vi "fgv_Video Recording Enable.vi"(9 "Function":T1, 11 "Video Recording Enabled":bool) -> (3 "Video Recording Enabled":bool)   [LabVIEW 2013]
uses:
  Typedefs/Read Write Enum.ctl
  Global Variables/General Globals.vi
panel:
  # "SUBROUTINE"
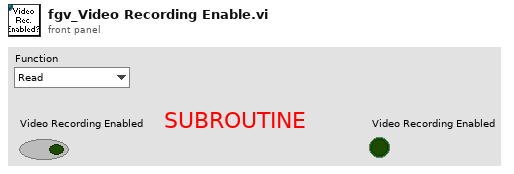
[diagram p1: front panel]
types:
  T1 = typedef "Read Write Enum.ctl" = enum16{"Read", "Write"}
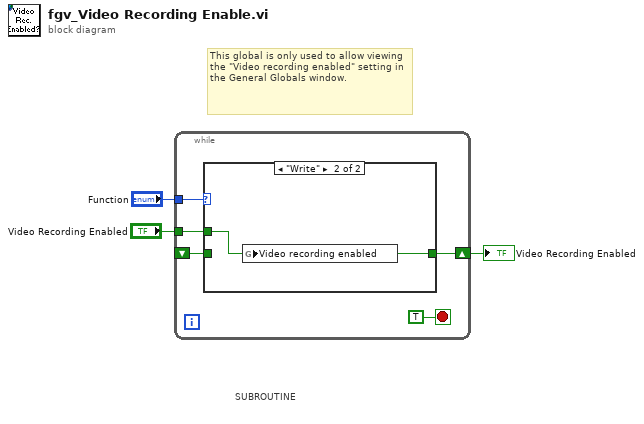
[diagram p0: block diagram]
diagram:
  # "SUBROUTINE"
  # "This global is only used to allow viewing the \"Video recording enabled\" setting in the General Globals window."
  n1 = while {
    tunnel: "Function" -> [w7]
    tunnel: "Video Recording Enabled" -> [w6]
    shift-right: [w5] -> w1
    shift-left: _ -> [w4]
    stop <- TRUE stop-if-true
    n2 = case shown="\"Write\"" w7 {
      tunnel: w6 -> [_ w10]
      tunnel: [w9 w10] -> w5
      tunnel: w4 -> [w9 _]
      frame "Read", Default {
      }
      frame "Write" {
        n3 = global write "General Globals.vi" "Video recording enabled"(w10) -> ()
      }
    }
  }
  "Video Recording Enabled" <- w1
